vi "disconnect.vi"(8 "error in (no error)":errorcluster, 11 "rethinkdb in":refnum<class "RethinkDB.lvclass">) -> (0 "error out":errorcluster, 3 "rethinkdb out":refnum<class "RethinkDB.lvclass">)   [LabVIEW 2017, in "rethinkdb.lvlib" / "RethinkDB.lvclass"]
uses:
  RethinkDB.lvclass
  RethinkDB.lvclass/RethinkDB.ctl
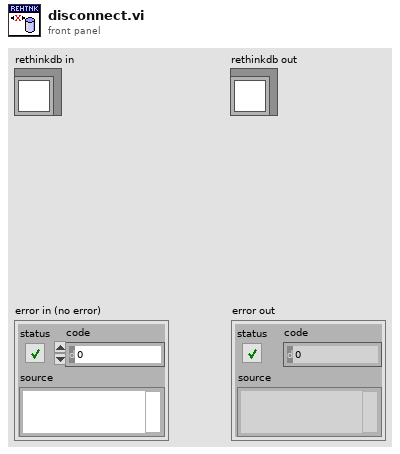
[diagram p1: front panel]
types:
  T1 = typedef "rethinkdb.lvlib/private.ctl" = cluster{"host":string, "port":u16, "ms_timeout":i32, "conn":refnum<k5>, "auth_key":string}
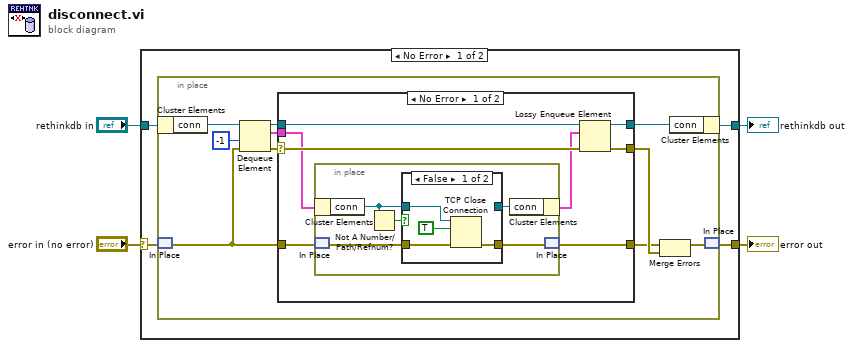
[diagram p0: block diagram]
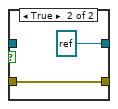
[diagram p2: hidden frame]
diagram:
  n1 = case shown="No Error" "error in (no error)" {
    selector: "error in (no error)" -> [w6 w42]
    tunnel: "rethinkdb in" -> [w8 w41]
    tunnel: [w5 w42] -> w3
    tunnel: [w7 w41] -> w1
    frame No Error {
      n2 = in-place {
        n3 = in-place-cluster #1(w8) -> ("conn"=w12:refnum<queue>)
        n4 = in-place-match #2(w6) -> (w10:errorcluster)
        n5 = Dequeue Element(queue=w12, timeout in ms (-1)=-1, error in (no error)=w10) -> (queue out=w17:refnum<queue>, element=w16:T1, error out=w15:errorcluster)  [unwired: 1 out]
        n6 = case shown="No Error" w15 {
          selector: w15 -> [w25 w40]
          tunnel: w17 -> [w26 w38]
          tunnel: w16 -> [w22 _]
          tunnel: [w24 w40] -> w14
          tunnel: w10 -> [w21 w39]
          tunnel: [w20 w39] -> w13
          tunnel: [w23 w38] -> w11
          frame No Error {
            n7 = in-place {
              n8 = in-place-cluster #3(w22) -> ("conn"=w30:refnum<k5>)
              n9 = in-place-match #4(w21) -> (w28:errorcluster)
              n10 = Not A Number/Path/Refnum?(number/path/refnum=w30) -> (NaN/Path/Refnum?=w31:bool)
              n11 = case shown="False" w31 {
                tunnel: w28 -> [w35 w37]
                tunnel: [w33 w37] -> w27
                tunnel: [_ refnum<k5> refnum ("conn")] -> w29
                tunnel: w30 -> [w32 _]
                frame False {
                  n12 = TCP Close Connection(connection ID=w32, abort (F)=TRUE, error in (no error)=w35) -> (error out=w33:errorcluster)  [unwired: 1 out]
                }
                frame True {
                }
              }
              n13 = in-place-cluster #3("conn"=w29) -> (w19:T1)
              n14 = in-place-match #4(w27) -> (w20:errorcluster)
            }
            n15 = Lossy Enqueue Element(queue=w26, element=w19, error in (no error)=w25) -> (queue out=w23:refnum<queue>, error out=w24:errorcluster)  [unwired: 2 out]
          }
          frame Error {
          }
        }
        n16 = Merge Errors(w13, w14) -> (w9:errorcluster)
        n17 = in-place-cluster #1("conn"=w11) -> (w7:refnum<class "RethinkDB.lvclass">)
        n18 = in-place-match #2(w9) -> (w5:errorcluster)
      }
    }
    frame Error {
    }
  }
  "error out" <- w3
  "rethinkdb out" <- w1
